vi "Read Heater I.vi"(8 "error in (no error)":errorcluster, 11 "LNG Boiling Results in":refnum<class "LNG Boiling Results.lvclass">) -> (0 "error out":errorcluster, 2 "Heater I":dbl, 3 "LNG Boiling Results out":refnum<class "LNG Boiling Results.lvclass">)   [LabVIEW 2019, in "Results.lvlib" / "LNG Boiling Results.lvclass"]
uses:
  LNG Boiling Results.lvclass
  LNG Boiling Results.lvclass/LNG Boiling Results.ctl
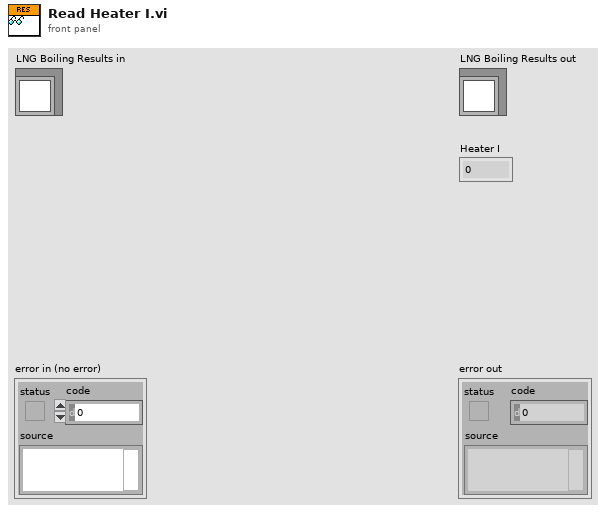
[diagram p1: front panel]
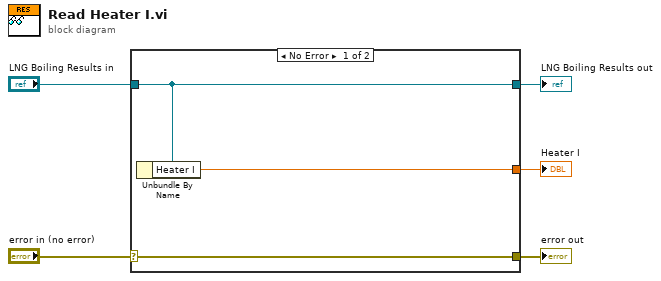
[diagram p0: block diagram]
diagram:
  n1 = case shown="No Error" "error in (no error)" {
    selector: "error in (no error)" -> [w8 w9]
    tunnel: [w8 w9] -> w4
    tunnel: [w7 w10] -> w2
    tunnel: "LNG Boiling Results in" -> [w7 w10]
    tunnel: [w6 _] -> w1
    frame No Error {
      n2 = Unbundle By Name(w7) -> ("Heater I"=w6:dbl)
    }
    frame Error {
    }
  }
  "error out" <- w4
  "LNG Boiling Results out" <- w2
  "Heater I" <- w1
